vi "ECAT Execute FoE Write.vi"(6 "Finish":bool=TRUE, 8 "error In":errorcluster, 9 "File Byte Array":u8[](array[numeric]), 11 "Slave Ref in":refnum<k21>) -> (0 "error Out":errorcluster, 3 "Slave Ref out":refnum<k21>)   [LabVIEW 2011, in "Scan Engine Custom Device.lvlib"]
uses:
  Scan Engine Custom Device.lvlib
  Program Files (x86)/National Instruments/LabVIEW 2011/resource/objmgr/IndComECAT.rc
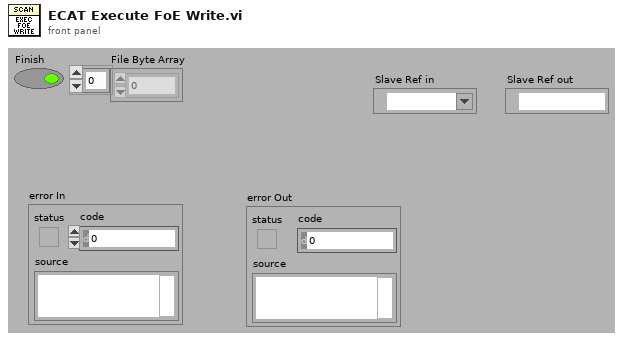
[diagram p1: front panel]
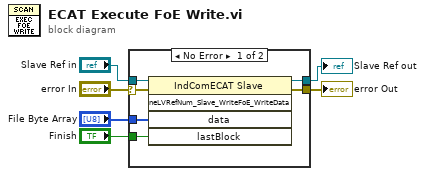
[diagram p0: block diagram]
diagram:
  n1 = case shown="No Error" "error In" {
    selector: "error In" -> [w10 w14]
    tunnel: "File Byte Array" -> [w12 _]
    tunnel: [w11 w14] -> w6
    tunnel: "Finish" -> [w9 _]
    tunnel: "Slave Ref in" -> [w8 w13]
    tunnel: [w7 w13] -> w1
    frame No Error {
      n2 = invoke class="IndComECAT Slave" method="neLVRefNum_Slave_WriteFoE_WriteData"(reference=w8, error in=w10, "data"=w12, "lastBlock"=w9) -> (reference out=w7:refnum<k21>, error out=w11:errorcluster)  [unwired: 1 in, 3 out]
    }
    frame Error {
    }
  }
  "error Out" <- w6
  "Slave Ref out" <- w1
